vi "Optical Pulse Sequence Generator.vi"(5 "ref?":bool, 6 "N Loop":i32=25000, 7 "Sig/Ref pause":dbl, 8 "AOM Rest time":dbl, 9 "Signal delay":dbl, 10 "APD signal width":dbl, 11 "AOM Pulse length":dbl=3e-07) -> (0 "Array":T1(array[cluster]), 3 "No. Instructions":i32)   [LabVIEW 2012]
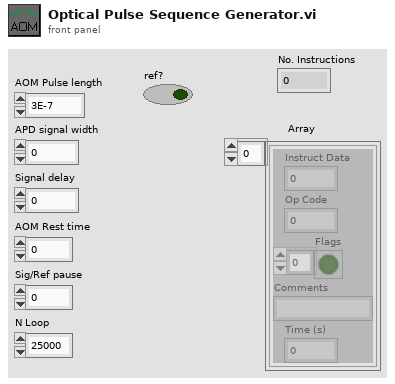
[diagram p1: front panel]
types:
  T1 = cluster{"Instruct Data":i32, "Op Code":i32, "Flags":bool[], "Comments":string, "Time (s)":dbl}[]
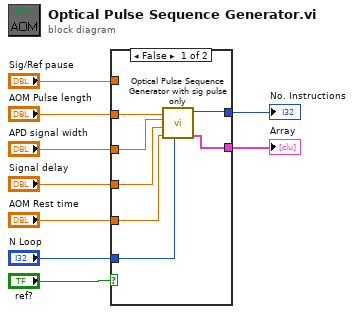
[diagram p0: block diagram]
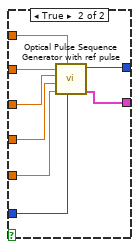
[diagram p2: hidden frame]
diagram:
  n1 = case shown="False" "ref?" {
    tunnel: "Sig/Ref pause" -> [_ w24]
    tunnel: "AOM Pulse length" -> [w14 w23]
    tunnel: "APD signal width" -> [w13 w22]
    tunnel: "Signal delay" -> [w12 w21]
    tunnel: "AOM Rest time" -> [w11 w20]
    tunnel: "N Loop" -> [w10 w19]
    tunnel: [w16 w18] -> w2
    tunnel: [w15 w17] -> w1
    frame False {
      n2 = call "Optical Pulse Sequence Generator with sig pulse only.vi"("N Loop"=w10, "AOM Rest time"=w11, "Signal delay"=w12, "APD signal width"=w13, "AOM Pulse length"=w14) -> ("Array"=w15:T1, "No. Instructions"=w16:i32)  [unwired: 5 in]
    }
    frame True {
      n3 = call "Optical Pulse Sequence Generator with ref pulse.vi"("N Loop"=w19, "Sig/Ref pause"=w24, "AOM Rest time"=w20, "Signal delay"=w21, "APD signal width"=w22, "AOM Pulse length"=w23) -> ("Array"=w17:T1, "No. Instructions"=w18:i32)  [unwired: 4 in]
    }
  }
  "Array" <- w1
  "No. Instructions" <- w2
